vi "Handle.vi"(7 "Event Actor in":refnum<class "Event Actor.lvclass">, 11 "Nominal Event State in":refnum<class "Nominal Event State.lvclass">) -> (2 "Destroy?":bool, 5 "Event Actor out":refnum<class "Event Actor.lvclass">)   [LabVIEW 2021, in "jettl.lvlib" / "Nominal Event State.lvclass"]
uses:
  Nominal Event State.lvclass
  Actor/Event Actor/Event Actor.lvclass
  eecdf29a-2c89-43b0-98ec-9b27f9f13fb9.vi/ff40df25-0e41-4205-825d-56c19dc320b6.vi
  <vilib>/Utility/Debug Log/Display.vi
  Nominal Event State.lvclass/Nominal Event State.ctl
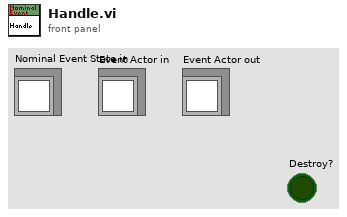
[diagram p1: front panel]
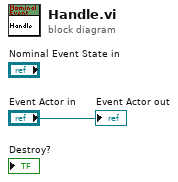
[diagram p0: block diagram]
diagram:
  "Event Actor out" <- "Event Actor in"
